vi "Restore Panel.vi"(6 "User":string, 8 "Error In":errorcluster, 10 "VI reference":refnum<vi>, 11 "Path (dialog)":path=path "C:/ProgramData/EPL/CFTS Defaults.ini") -> (0 "error out":errorcluster)   [LabVIEW 2020]
doc: "Attempt to restore panel controls from a file.\n\nFreeware from Moore Good Ideas, www.mooregoodideas.com. Do not remove this line.\ndavid@mooregoodideas.com"
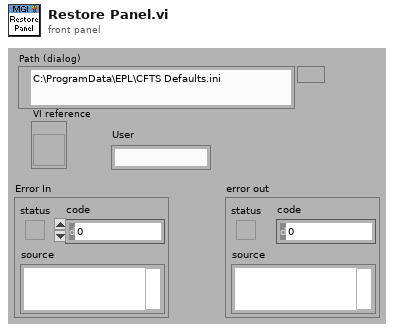
[diagram p1: front panel]
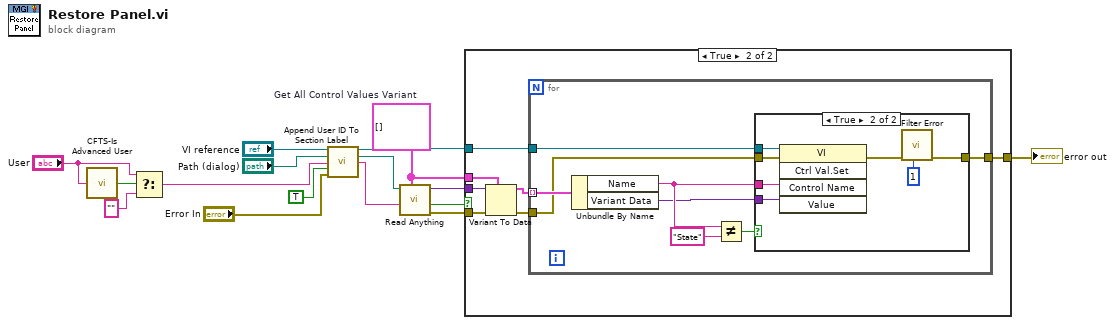
[diagram p0: block diagram]
diagram:
  w16 = cluster{"Name":string, "Variant Data":variant}[] []  # Get All Control Values Variant
  n1 = call "CFTS-Is Advanced User.vi"("Experimenter"="User") -> ("Advanced user"=w5:bool)
  n2 = Select(t="User", s=w5, f="") -> (s? t:f=w2:string)
  n3 = call "Append User ID To Section Label.vi"("VI reference"="VI reference", "Path (dialog)"="Path (dialog)", "User"=w2, "Section must exist?"=TRUE, "error in (no error)"="Error In") -> ("VI reference (thru)"=w7:refnum<vi>, "Path (thru)"=w9:path, "Section Name"=w1:string)  [unwired: 7 in, 1 out]
  n4 = call "Read Anything.vi"("Type of Anything"=w16, "Section Name (Name of \"Type of Anything\")"=w1, "Path (dialog)"=w9) -> ("Error Out"=w14:errorcluster, "Found?"=w12:bool, "Anything"=w15:variant)  [unwired: 1 in, 5 out]
  n5 = case shown="True" w12 {
    tunnel: w16 -> [_ w22]
    tunnel: w15 -> [_ w21]
    tunnel: w14 -> [w17 w20]
    tunnel: w7 -> [_ w19]
    tunnel: [w17 w18] -> w13
    frame False {
    }
    frame True {
      n6 = Variant To Data(error in=w20, type=w22, Variant=w21) -> (data=w23:cluster{"Name":string, "Variant Data":variant}[], error out=w24:errorcluster)
      n7 = for {
        tunnel: w23 -> [w32] mode=indexing
        tunnel: w19 -> [w31]
        tunnel: w24 -> [w30]
        tunnel: [w26] -> w18
        n8 = Unbundle By Name(w32) -> ("Name"=w28:string, "Variant Data"=w25:variant)
        n9 = Not Equal?(x=w28, y="State") -> (x != y?=w27:bool)
        n10 = case shown="True" w27 {
          tunnel: w25 -> [_ w40]
          tunnel: w31 -> [_ w39]
          tunnel: w30 -> [w33 w38]
          tunnel: w28 -> [_ w37]
          tunnel: [w33 w35] -> w26
          frame False {
          }
          frame True {
            n11 = invoke class="VI" method="Ctrl Val.Set"(reference=w39, error in=w38, "Control Name"=w37, "Value"=w40) -> (error out=w36:errorcluster)  [unwired: 1 in, 4 out]
            n12 = call "Filter Error.vi"("error in (no error)"=w36, "code to ignore"=1) -> ("error out"=w35:errorcluster)  [unwired: 9 in]
          }
        }
      }
    }
  }
  "error out" <- w13
